vi "Generate IMD Multitone Waveform.vi"(6 "hardware commands sync queue":T2, 8 "error in":errorcluster, 9 "measurement configuration":T1={"Full scale range"=2.825, "Channel name"="", "Analog source resource name"="", "IMD standard"=enum."SMPTE (60 Hz, 7000 Hz, 4:1)", "Low frequency"=0.0, "High frequency"=0.0, "Amplitude ratio"=0.0, "Amplitude"=0.0, "Protocol capture resource name"="", "Data line"=0, "Channel"=0, "Sample rate"=44100.0, "Measurement duration"=0.1, "Frame sync edge for Channel 0"=enum."Falling", "Channel count per frame"=2, "Channel length"=32, "Bit depth"=24, "Channel 0 offset"=1, "Endianness"=enum."MSB First", "Data Justification"=enum."Left Justified", "Frame length"=64, "Frame sync pulse width"=32, "Bit clock edge  sync"=enum."Falling"}, 10 "Sample rate":dbl, 11 "DSG task in":refnum<k21>) -> (0 "error out":errorcluster, 3 "DSG task out":refnum<k21>)   [LabVIEW 2021, in "IMD_Audio ADC.lvlib"]
uses:
  IMD_Audio ADC.lvlib
  shared/controls/Sync Commands Queue Ref.ctl
  shared/controls/Sync Commands.ctl
  Measurement Configuration.ctl
  <vilib>/addons/_NISVFA/_Generation/Signal Generation/SV Signal/sv_System Timing Model.ctl
  <vilib>/DAQmx/write.llb/DAQmx Write (Analog 1D Wfm NChan NSamp).vi
  <vilib>/addons/_NISVFA/_Generation/Signal Generation/SV Multitone/SV Multitone.lvclass
  C:/Program Files/National Instruments/LabVIEW 2021/vi.lib/addons/_NISVFA/_Generation/Signal Generation/SV Signal/SV Signal.lvclass
  <vilib>/addons/_NISVFA/_Generation/Signal Generation/SV Multitone/Configure Multitone (Custom).vi
  <vilib>/addons/_NISVFA/_Generation/Signal Generation/SV Signal/Write Sample Rate.vi
  <vilib>/addons/_NISVFA/_Generation/Signal Generation/SV Signal/Write System Timing Model.vi
  <vilib>/addons/_NISVFA/_Generation/Signal Generation/SV Signal/Write Ramp Parameters.vi
  <vilib>/DAQmx/miscellaneous.llb/DAQmx Fill In Error Info.vi
  shared/controls/Audio ADC Controls.lvlib
  <vilib>/addons/_NISVFA/_Generation/Signal Generation/SV Signal/SV Signal.lvclass
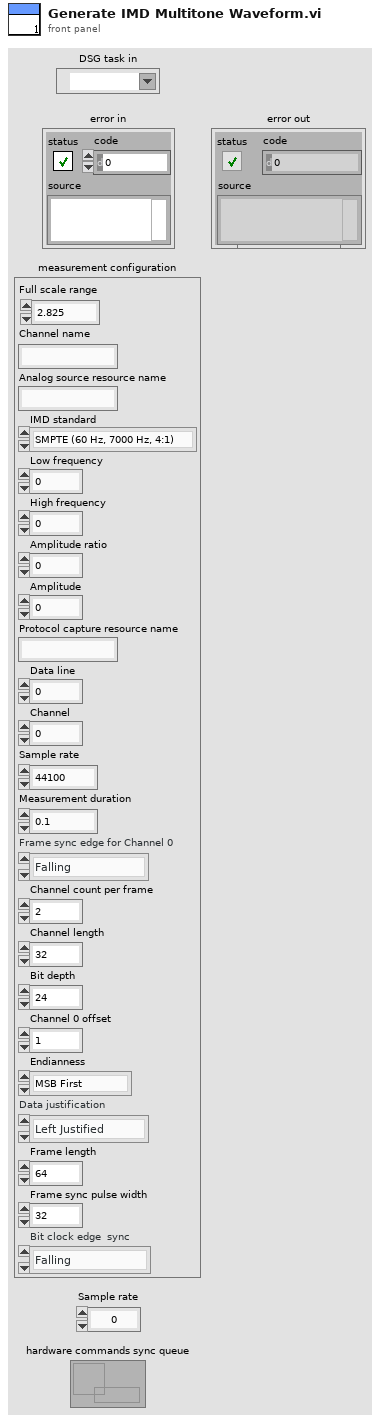
[diagram p1: front panel]
types:
  T1 = typedef "IMD_Audio ADC.lvlib/Measurement Configuration.ctl" = cluster{"Full scale range":dbl, "Channel name":string, "Analog source resource name":string, "IMD standard":enum16{"SMPTE (60 Hz, 7000 Hz, 4:1)", "DIN (250 Hz, 8000 Hz, 4:1)", "CCIF (11 kHz, 12 kHz, 1:1)", "CCIF (19 kHz, 20 kHz, 1:1)", "Custom"}, "Low frequency":dbl, "High frequency":dbl, "Amplitude ratio":dbl, "Amplitude":dbl, "Protocol capture resource name":string, "Data line":u32, "Channel":u32, "Sample rate":dbl, "Measurement duration":dbl, "Frame sync edge for Channel 0":enum32{"Rising", "Falling"}, "Channel count per frame":u32, "Channel length":u32, "Bit depth":u32, "Channel 0 offset":u32, "Endianness":enum32{"MSB First", "LSB First"}, "Data Justification":enum32{"Left Justified", "Right Justified"}, "Frame length":u32, "Frame sync pulse width":u32, "Bit clock edge  sync":enum32{"Rising", "Falling"}}
  T2 = typedef "Audio ADC Controls.lvlib/Sync Commands Queue Ref.ctl" = refnum<queue>
  T3 = cluster{"profile":enum16{"Linear", "Half cosine"}, "durations [s]":cluster{"ramp-up":dbl, "transition":dbl, "ramp-down":dbl}}
  T4 = typedef "audio adc controls.lvlib/Sync Commands.ctl" = enum16{"NoAction", "GenerationStarted", "AcquisitionCompleted", "GenerationErrored"}
  T5 = typedef "SV Signal.lvclass/sv_System Timing Model.ctl" = i64
  T6 = enum16{"SMPTE (60 Hz, 7000 Hz, 4:1)", "DIN (250 Hz, 8000 Hz, 4:1)", "CCIF (11 kHz, 12 kHz, 1:1)", "CCIF (19 kHz, 20 kHz, 1:1)", "Custom"}
  T7 = typedef "Audio ADC Controls.lvlib/Sync Commands.ctl" = enum16{"NoAction", "GenerationStarted", "AcquisitionCompleted", "GenerationErrored"}
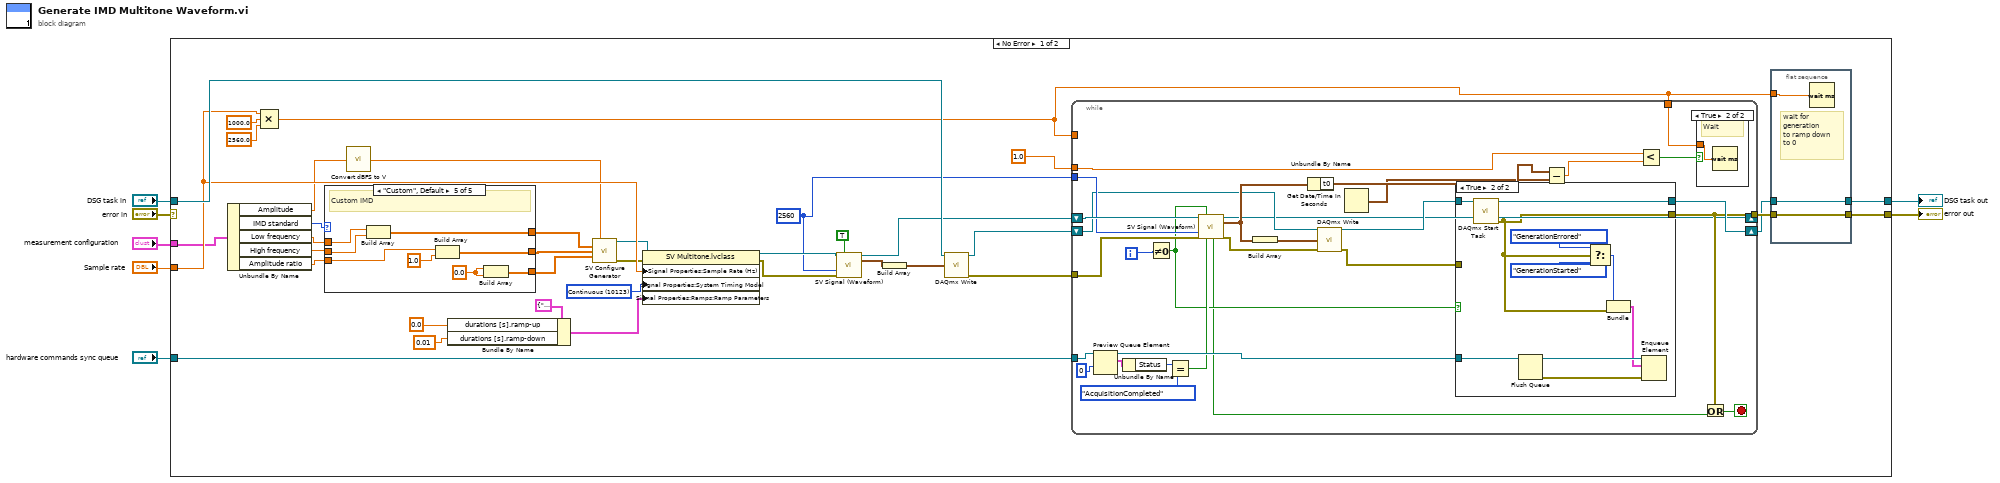
[diagram p0: block diagram]
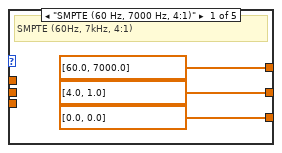
[diagram p2: hidden frame]
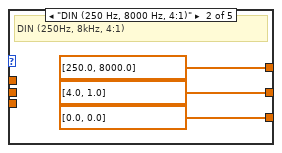
[diagram p3: hidden frame]
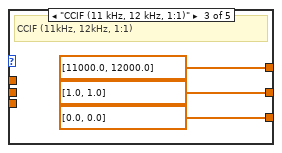
[diagram p4: hidden frame]
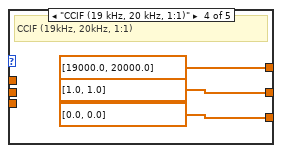
[diagram p5: hidden frame]
diagram:
  n1 = case shown="No Error" "error in" {
    selector: "error in" -> [_ w111]
    tunnel: [w44 w110] -> w6
    tunnel: [w43 w111] -> w5
    tunnel: "DSG task in" -> [w41 w110]
    tunnel: "hardware commands sync queue" -> [w42 _]
    tunnel: "Sample rate" -> [w40 _]
    tunnel: "measurement configuration" -> [w39 _]
    frame No Error {
      w10 = 2560 ("samples")
      w27 = T5 10123 items=["Finite"=10178, "-"=-1, "Continuous"=10123, "-"=-2, "Settled"=110123, "Averaged"=210123, "Discrete Sweep"=310123, "Continuous Sweep"=410123] ("System Timing Model")
      n2 = Unbundle By Name(w39) -> ("Amplitude"=w30:dbl, "IMD standard"=w36:T6, "Low frequency"=w35:dbl, "High frequency"=w34:dbl, "Amplitude ratio"=w33:dbl)
      n3 = Compound Arithmetic op=MULTIPLY(w40, 1000.0 ("value"), 2560.0 ("value")) -> (w8:dbl)
      n4 = case shown="\"Custom\", Default" w36 {
        tunnel: [dbl[] [60.0, 7000.0] ("source settings.frequencies") dbl[] [250.0, 8000.0] ("source settings.frequencies") dbl[] [11000.0, 12000.0] ("source settings.frequencies") dbl[] [19000.0, 20000.0] ("source settings.frequencies") w62] -> w21
        tunnel: [dbl[] [4.0, 1.0] ("source settings.frequencies") dbl[] [4.0, 1.0] ("source settings.frequencies") dbl[] [1.0, 1.0] ("source settings.frequencies") dbl[] [1.0, 1.0] ("source settings.frequencies") w61] -> w20
        tunnel: [dbl[] [0.0, 0.0] ("source settings.frequencies") dbl[] [0.0, 0.0] ("source settings.frequencies") dbl[] [0.0, 0.0] ("source settings.frequencies") dbl[] [0.0, 0.0] ("source settings.frequencies") w60] -> w19
        tunnel: w35 -> [_ _ _ _ w59]
        tunnel: w34 -> [_ _ _ _ w58]
        tunnel: w33 -> [_ _ _ _ w57]
        frame "SMPTE (60 Hz, 7000 Hz, 4:1)" {
          # "SMPTE (60Hz, 7kHz, 4:1)"
        }
        frame "DIN (250 Hz, 8000 Hz, 4:1)" {
          # "DIN (250Hz, 8kHz, 4:1)"
        }
        frame "CCIF (11 kHz, 12 kHz, 1:1)" {
          # "CCIF (11kHz, 12kHz, 1:1)"
        }
        frame "CCIF (19 kHz, 20 kHz, 1:1)" {
          # "CCIF (19kHz, 20kHz, 1:1)"
        }
        frame "Custom", Default {
          w63 = 0.0 ("element")
          # "Custom IMD"
          n5 = Build Array(w59, w58) -> (w62:dbl[])
          n6 = Build Array(w57, 1.0 ("element")) -> (w61:dbl[])
          n7 = Build Array(w63, w63) -> (w60:dbl[])
        }
      }
      n8 = call "Convert dBFS to V.vi"("Amplitude (dBFS)"=w30) -> ("Amplitude (V)"=w24:dbl)
      n9 = Bundle By Name(cluster=T3 {"profile"=enum."Linear", "durations [s]"={"ramp-up"=0.0, "transition"=0.0, "ramp-down"=0.0}} ("Ramp Parameters:All Elements"), "durations [s].ramp-up"=0.0, "durations [s].ramp-down"=0.01) -> (w26:T3)
      n10 = call-poly <vilib>:"SV Configure Generator.vi"("overall amplitude"=w24, "frequencies [Hz]"=w21, "amplitudes"=w20, "phases [deg]"=w19) -> ("signal configuration"=w23:refnum<class "SV Multitone.lvclass">, "error out"=w22:errorcluster)  [unwired: 9 in, 1 out]
      n11 = property class="SV Multitone.lvclass"(reference=w23, error in=w22, "Signal Properties:Sample Rate (Hz)"=w40, "Signal Properties:System Timing Model"=w27, "Signal Properties:Ramps:Ramp Parameters"=w26) -> (reference out=w18:refnum<class "SV Multitone.lvclass">, error out=w16:errorcluster)
      n12 = call-dynamic "SV Signal (Waveform).vi"("signal configuration"=w18, "reset"=TRUE, "samples"=w10, "error in (no error)"=w16) -> ("signal configuration"=w12:refnum<class "SV Multitone.lvclass">, "output waveform"=w15:waveform(dbl))  [unwired: 6 in, 4 out]
      n13 = Build Array(w15) -> (w14:waveform(dbl)[])
      n14 = call-poly <vilib>:"DAQmx Write.vi"("task/channels in"=w41, "data"=w14) -> ("task out"=w13:refnum<k21>, "error out"=w11:errorcluster)  [unwired: 11 in, 1 out]
      n15 = while {
        shift-right: [w68] -> _
        shift-left: w12 -> [w83]
        shift-right: [w91] -> w37
        shift-left: w13 -> [w80]
        tunnel: [w88] -> w38
        tunnel: w42 -> [w95]
        tunnel: w11 -> [w81]
        tunnel: w10 -> [w82]
        tunnel: 1.0 -> [w71]
        tunnel: w8 -> [_]
        tunnel: w8 -> [w69]
        i -> [w84]
        stop <- w96 stop-if-true
        n16 = Preview Queue Element(queue=w95, timeout in ms (-1)=0) -> (queue out=w92:T2, element=w90:cluster{"Status":T7, "Error":errorcluster})  [unwired: 1 in, 2 out]
        n17 = Unbundle By Name(w90) -> ("Status"=w89:T7)
        n18 = Not Equal To 0?(x=w84) -> (x != 0?=w77:bool)
        n19 = Equal?(x=w89, y=Sync_Commands."AcquisitionCompleted") -> (x = y?=w78:bool)
        n20 = call-dynamic "SV Signal (Waveform).vi"("signal configuration"=w83, "reset"=w77, "samples"=w82, "error in (no error)"=w81, "stop"=w78) -> ("signal configuration"=w68:refnum<class "SV Multitone.lvclass">, "output waveform"=w87:waveform(dbl), "done"=w75:bool, "error out"=w85:errorcluster)  [unwired: 5 in, 2 out]
        n21 = Build Array(w87) -> (w86:waveform(dbl)[])
        n22 = Unbundle By Name(w87) -> ("t0"=w74:timestamp)
        n23 = call-poly <vilib>:"DAQmx Write.vi"("task/channels in"=w80, "data"=w86, "error in"=w85) -> ("task out"=w79:refnum<k21>, "error out"=w76:errorcluster)  [unwired: 10 in, 1 out]
        n24 = Get Date/Time In Seconds() -> (seconds since 1Jan1904=w73:timestamp)
        n25 = case shown="True" w77 {
          tunnel: w92 -> [_ w109]
          tunnel: [w99 w107] -> w91
          tunnel: [w98 w102] -> w88
          tunnel: w79 -> [w99 w100]
          tunnel: w76 -> [w98 _]
          frame False {
          }
          frame True {
            n26 = call <vilib>:"DAQmx Start Task.vi"("task/channels in"=w100) -> ("task out"=w107:refnum<k21>, "error out"=w102:errorcluster)  [unwired: 13 in]
            n27 = Flush Queue(queue=w109) -> (queue out=w108:T2, error out=w106:errorcluster)  [unwired: 1 in, 1 out]
            n28 = Select(t=Sync_Commands."GenerationErrored" ("element"), s=w102, f=Sync_Commands."GenerationStarted" ("element")) -> (s? t:f=w103:T4)
            n29 = Bundle("element"=w103, "error out"=w102) -> (w101:cluster{"element":T4, "error out":errorcluster})  [unwired: 1 in]
            n30 = Enqueue Element(queue=w108, element=w101, error in (no error)=w106) -> ()  [unwired: 1 in, 3 out]
          }
        }
        n31 = Subtract(x=w74, y=w73) -> (x-y=w72:dbl)
        n32 = Less?(x=w71, y=w72) -> (x < y?=w70:bool)
        n33 = case shown="True" w70 {
          tunnel: w69 -> [_ w97]
          frame False {
          }
          frame True {
            # "Wait"
            n34 = Wait (ms)(milliseconds to wait=w97) -> ()  [unwired: 1 out]
          }
        }
        n35 = Or(x=w88, y=w75) -> (x .or. y?=w96:bool)
      }
      n36 = flat-sequence {
        tunnel: w38 -> [w66]
        tunnel: w37 -> [w67]
        tunnel: [w67] -> w44
        tunnel: [w66] -> w43
        tunnel: w8 -> [w65]
        frame #0 {
          # "wait for\ngeneration\nto ramp down\nto 0"
          n37 = Wait (ms)(milliseconds to wait=w65) -> ()  [unwired: 1 out]
        }
      }
    }
    frame Error {
    }
  }
  "DSG task out" <- w6
  "error out" <- w5
